vi "VisionSystem.vi"() -> ()   [LabVIEW 2025]
panel:
  out "Vision/Cam1Orientation 4":dbl caption="Cam 1 Yaw" format="%11.2f"
  out "Vision/CamZ 4":dbl caption="Cam 1 Z" format="%11.2f"
  out "Vision/Cam1Y 4":dbl caption="Cam 1 Y" format="%11.2f"
  out "Vision/Cam1Count 4":dbl caption="Cam1 Count" format="%13.0f"
  out "Vision/Cam1X 4":dbl caption="Cam 1 X" format="%11.2f"
  out "Vision/Cam1Orientation 3":dbl caption="Cam 1 Yaw" format="%11.2f"
  out "Vision/CamZ 3":dbl caption="Cam 1 Z" format="%11.2f"
  out "Vision/Cam1Y 3":dbl caption="Cam 1 Y" format="%11.2f"
  out "Vision/Cam1Count 3":dbl caption="Cam1 Count" format="%13.0f"
  out "Vision/Cam1X 3":dbl caption="Cam 1 X" format="%11.2f"
  out "Vision/Cam1Orientation 2":dbl caption="Cam 1 Yaw" format="%11.2f"
  out "Vision/CamZ 2":dbl caption="Cam 1 Z" format="%11.2f"
  out "Vision/Cam1Y 2":dbl caption="Cam 1 Y" format="%11.2f"
  out "Vision/Cam1Count 2":dbl caption="Cam1 Count" format="%13.0f"
  out "Vision/Cam1X 2":dbl caption="Cam 1 X" format="%11.2f"
  out "Vision/Cam1Orientation":dbl caption="Cam 1 Yaw" format="%11.2f"
  out "Vision/CamZ":dbl caption="Cam 1 Z" format="%11.2f"
  out "Vision/Cam1Y":dbl caption="Cam 1 Y" format="%11.2f"
  out "Vision/Cam1Count":dbl caption="Cam1 Count" format="%13.0f"
  out "Vision/Cam1X":dbl caption="Cam 1 X" format="%11.2f"
  # "VISION"
  # "Cam 1"
  # "Cam 2"
  # "Cam 3"
  # "Cam 4"
  # "Count"
  # "X"
  # "Y"
  # "Z"
  # "Yaw"
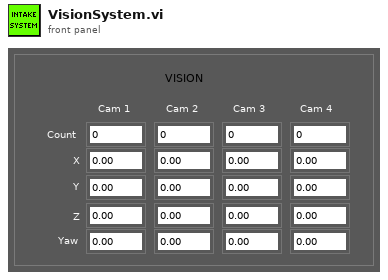
[diagram p1: front panel]
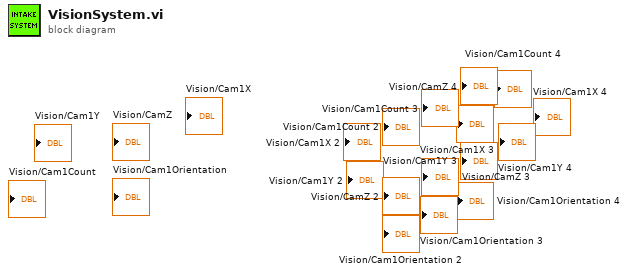
[diagram p0: block diagram]
diagram:
